vi "make_sd_histogram.vi"(11 "waveform":waveform(dbl)) -> (0 "Százalékos hiba [%]":dbl, 1 "Konfidencia intervallum [g]":dbl, 2 "Szórás [g]":dbl, 3 "Középérték [g]":dbl, 4 "standard deviation":dbl format="%0.2f", 8 "Empirikus sûrûségfüggvény":cluster{"X Values":dbl[], dbl[]}(graph), 9 "Gyakoriság hisztogram":T1(graph))   [LabVIEW 2019]
uses:
  <vilib>/Analysis/NI_AALBase.lvlib
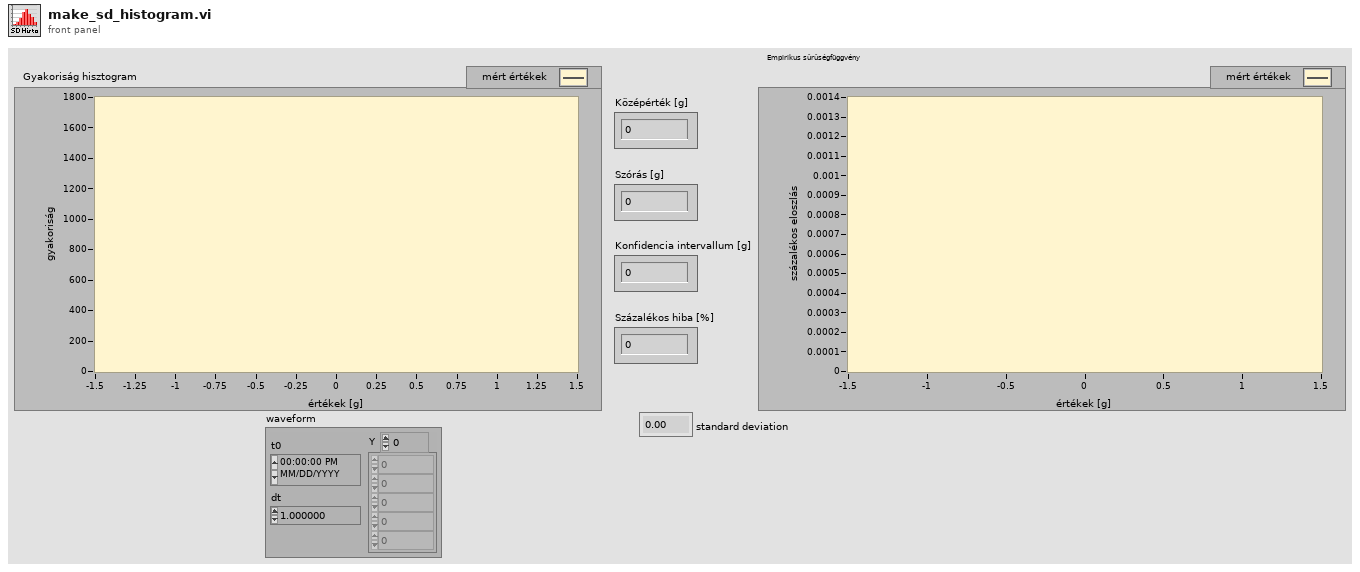
[diagram p1: front panel]
types:
  T1 = cluster{"X Values":dbl[], "Histogram: h(x)":i32[]}
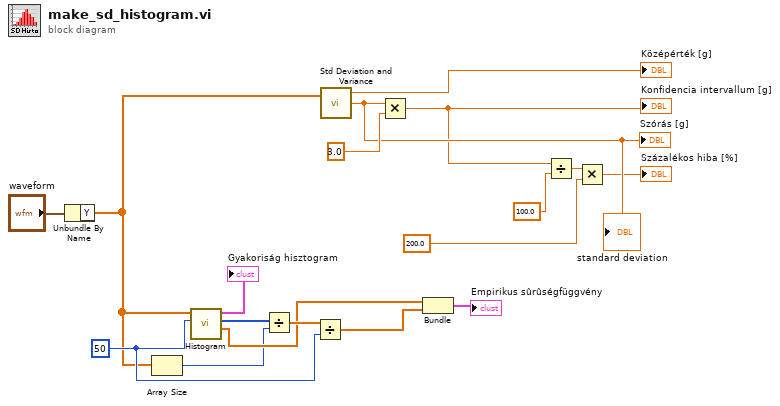
[diagram p0: block diagram]
diagram:
  w11 = 50
  n1 = Unbundle By Name("waveform") -> ("Y"=w1:dbl[])
  n2 = Array Size(array=w1) -> (size(s)=w7:i32)
  n3 = call <vilib>:"Histogram.vi"("intervals"=w11, "X"=w1) -> ("X Values"=w13:dbl[], "Histogram: h(x)"=w17:i32[], "Histogram Graph"=→"Gyakoriság hisztogram":T1)  [unwired: 6 in, 1 out]
  n4 = Divide(x=w17, y=w7) -> (x/y=w16:dbl[])
  n5 = Divide(x=w16, y=w11) -> (x/y=w14:dbl[])
  n6 = call <vilib>:"Std Deviation and Variance.vi"("X"=w1) -> ("mean"=→"Középérték [g]":dbl, "standard deviation"=w15:dbl)  [unwired: 1 in, 1 out]
  "Szórás [g]" <- w15
  "standard deviation" <- w15
  n7 = Multiply(x=w15, y=3.0) -> (x*y=w3:dbl)
  "Konfidencia intervallum [g]" <- w3
  n8 = Bundle("X Values"=w13, w14) -> (→"Empirikus sûrûségfüggvény":cluster{"X Values":dbl[], dbl[]})  [unwired: 1 in]
  n9 = Divide(x=w3, y=100.0) -> (x/y=w8:dbl)
  n10 = Multiply(x=w8, y=200.0) -> (x*y=→"Százalékos hiba [%]":dbl)
